vi "Read Response.vi"(8 "error in (no error)":errorcluster, 11 "HttpResponseMessage in":refnum<class "HttpResponseMessage.lvclass">) -> (0 "error out":errorcluster, 1 "HttpContent out":refnum<class "HttpContent.lvclass">, 2 "HTTPHeaders_NET out":refnum<class "HttpHeaders_Response.lvclass">, 3 "HttpResponseMessage out":refnum<class "HttpResponseMessage.lvclass">, 4 "Timeout":bool, 5 "StatusCode":i32(ring)=100 items=["Continue"=100, "SwitchingProtocols"=101, "OK"=200, "Created"=201, "Accepted"=202, "NonAuthoritativeInformation"=203, "NoContent"=204, "ResetContent"=205, "PartialContent"=206, "MultipleChoices, Ambiguous"=300, "MovedPermanently, Moved"=301, "Found, Redirect"=302, "SeeOther, RedirectMethod"=303, "NotModified"=304, "UseProxy"=305, "Unused"=306, "TemporaryRedirect, RedirectKeepVerb"=307, "BadRequest"=400, "Unauthorized"=401, "PaymentRequired"=402, "Forbidden"=403, "NotFound"=404, "MethodNotAllowed"=405, "NotAcceptable"=406, "ProxyAuthenticationRequired"=407, "RequestTimeout"=408, "Conflict"=409, "Gone"=410, "LengthRequired"=411, "PreconditionFailed"=412, "RequestEntityTooLarge"=413, "RequestUriTooLong"=414, "UnsupportedMediaType"=415, "RequestedRangeNotSatisfiable"=416, "ExpectationFailed"=417, "UpgradeRequired"=426, "InternalServerError"=500, "NotImplemented"=501, "BadGateway"=502, "ServiceUnavailable"=503, "GatewayTimeout"=504, "HttpVersionNotSupported"=505], 6 "ReasonPhrase":string)   [LabVIEW 2018, in "HttpClient_NET.lvlib" / "HttpResponseMessage.lvclass"]
doc: "<b> </b> <b> </b>\nHttpClient_NET\nJustin Young - Viviota\nCopyright (c) 2021\nLicense: BSD"
uses:
  HttpResponseMessage.lvclass
  HttpHeaders_response/HttpHeaders_Response.lvclass
  HttpContent/HttpContent.lvclass
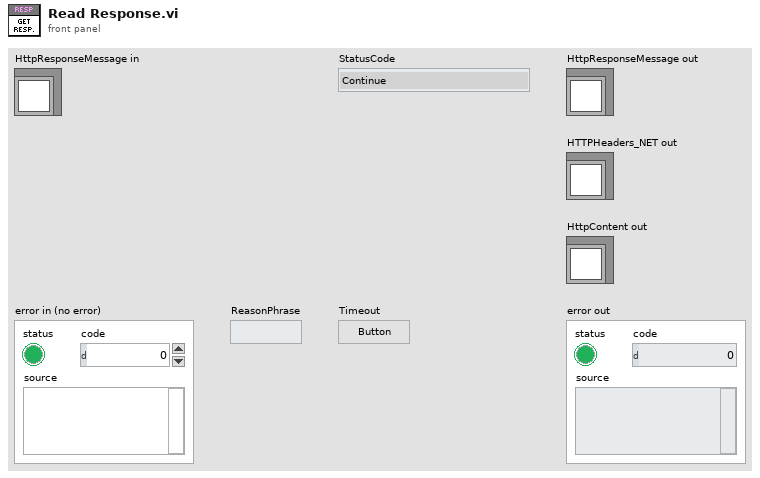
[diagram p1: front panel]
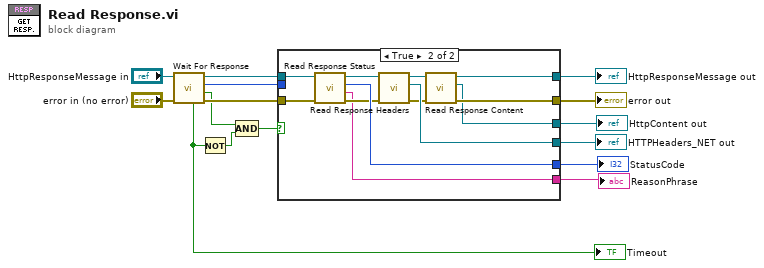
[diagram p0: block diagram]
diagram:
  n1 = call "Wait For Response.vi"("error in (no error)"="error in (no error)", "HttpResponseMessage in"="HttpResponseMessage in") -> ("error out"=w10:errorcluster, "TaskIsCompleted"=w7:bool, "TaskStatus"=w2:i32, "HttpResponseMessage out"=w9:refnum<class "HttpResponseMessage.lvclass">, "TaskTimeout"=w5:bool)  [unwired: 5 in]
  "Timeout" <- w5
  n2 = Not(x=w5) -> (.not. x?=w6:bool)
  n3 = Compound Arithmetic op=AND(w7, w6) -> (w4:bool)
  n4 = case shown="True" w4 {
    tunnel: [w16 w29] -> w15
    tunnel: [_ w28] -> w3
    tunnel: [w17 w27] -> w13
    tunnel: [_ w26] -> w12
    tunnel: [_ w25] -> w11
    tunnel: w10 -> [w16 w20]
    tunnel: w9 -> [w17 w19]
    tunnel: w2 -> [_ _]
    tunnel: [_ w18] -> w1
    frame False {
    }
    frame True {
      n5 = call "Read Response Status.vi"("error in (no error)"=w20, "HttpResponseMessage in"=w19) -> ("error out"=w22:errorcluster, "ReasonPhrase"=w18:string, "StatusCode"=w28:i32, "HttpResponseMessage out"=w21:refnum<class "HttpResponseMessage.lvclass">)  [unwired: 4 in, 2 out]
      n6 = call "Read Response Headers.vi"("error in (no error)"=w22, "HttpResponseMessage in"=w21) -> ("error out"=w24:errorcluster, "HTTPHeaders_NET out"=w26:refnum<class "HttpHeaders_Response.lvclass">, "HttpResponseMessage out"=w23:refnum<class "HttpResponseMessage.lvclass">)  [unwired: 7 in]
      n7 = call "Read Response Content.vi"("error in (no error)"=w24, "HttpResponseMessage in"=w23) -> ("error out"=w29:errorcluster, "HttpContent out"=w25:refnum<class "HttpContent.lvclass">, "HttpResponseMessage out"=w27:refnum<class "HttpResponseMessage.lvclass">)  [unwired: 7 in]
    }
  }
  "error out" <- w15
  "HttpResponseMessage out" <- w13
  "HTTPHeaders_NET out" <- w12
  "HttpContent out" <- w11
  "StatusCode" <- w3
  "ReasonPhrase" <- w1
